vi "PH_SSAC.Draw GUI Image.vi"(0 "i ref in":refnum<vi>, 5 "error in":errorcluster) -> (14 "i ref out":refnum<vi>, 19 "error out":errorcluster)   [LabVIEW 2014, in "PH_SSAC.lvlib"]
doc: "This VI draws the image to the GUI."
uses:
  PH_SSAC.lvlib
  PH_Basics/PH_Img_BaseClass/PH_Img_BaseClass.lvlib
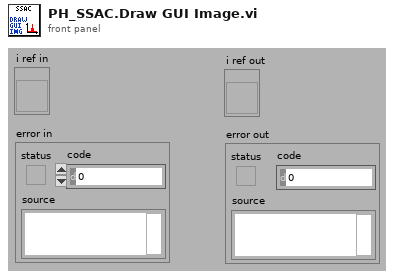
[diagram p1: front panel]
types:
  T1 = typedef "PH_SSAC.lvlib/PH_SSAC.i attribute.ctl" = cluster{"GUI Refs":cluster{"Delete":refnum<vi>, "Global On":refnum<vi>, "Cam Source":refnum<vi>, "Frame Main Signal":refnum<vi>, "Frame Background":refnum<vi>, "dt (Gauss smooth)":refnum<vi>, "Calibration Factor":refnum<vi>, "Background acquire":refnum<vi>, "Threshold":refnum<vi>, "Time evolution of mean pulse duration":refnum<vi>, "Mean Pulse Duration":refnum<vi>, "Main signal":refnum<vi>, "Current Pulse Duration":refnum<vi>, "Processed":refnum<vi>, "Saturation":refnum<vi>, "# for Average":refnum<vi>, "Position":refnum<vi>, "BG Status":refnum<vi>, "Save BG data":refnum<vi>, "Read BG Data":refnum<vi>, "Background Calibration Data":refnum<vi>}, "Images":cluster{"OP Image":T2, "GUI Image":T2, "PSDB Image":T2}, "Global On?":bool, "Frame Main":cluster{"x":u32, "dx":u32, "y":u32, "dy":u32}, "Frame Background":cluster{"x":u32, "dx":u32, "y":u32, "dy":u32}, "dt [fs]":dbl, "Calibration Factor [fs/pixel]":dbl, "Threshold":dbl, "Time evolution of mean pulse duration [fs]":dbl[], "Main Signal":cluster{"Time for Main":dbl[], "Signal":dbl[]}, "Processed":bool, "Current Pulse Duration [fs]":dbl, "# for Average":i32, "Position":i32, "Pulse Durations [fs]":dbl[], "BG":cluster{"Acquire?":bool, "Background Calibration Data":T3, "Save Data":bool}}
  T2 = typedef "IMAQ Image.ctl" = refnum<image>
  T3 = typedef "PH_SSAC.lvlib/PH_SSAC.Background Data.ctl" = cluster{"Date":string, "Time":string, "Frame Main":cluster{"x":u32, "dx":u32, "y":u32, "dy":u32}, "dt [fs]":dbl, "Calibration Factor [fs/pixel]":dbl, "Signal":dbl[], "Frame Background":cluster{"x":u32, "dx":u32, "y":u32, "dy":u32}}
  T4 = cluster{"Left":i32, "Top":i32, "Right":i32, "Bottom":i32}
  T5 = typedef "PH_Img_BaseClass.lvlib/PH_Img_BaseClass.i attribute.ctl" = cluster{"GUI Refs":T6, "Timeout Image [ms]":i32, "Default Periodic Period [ms]":i32, "Camera":cluster{"Instancename":string, "Notifier":refnum<notifier>}, "Palette":T7, "Cam Settings":cluster{"Cam ID":string, "Gain":dbl, "Brightness":dbl, "Shutter":dbl, "Cam Info Failure":bool, "Mode":i32}}
  T6 = typedef "PH_Img_BaseClass.lvlib/PH_Img_BaseClass.GUI Refs.ctl" = cluster{"Timeout":refnum<vi>, "Image":refnum<vi>, "Palette":refnum<vi>, "Timeout Set":refnum<vi>}
  T7 = typedef "PH_Img_BaseClass.lvlib/PH_Img_BaseClass.Palette.ctl" = i32
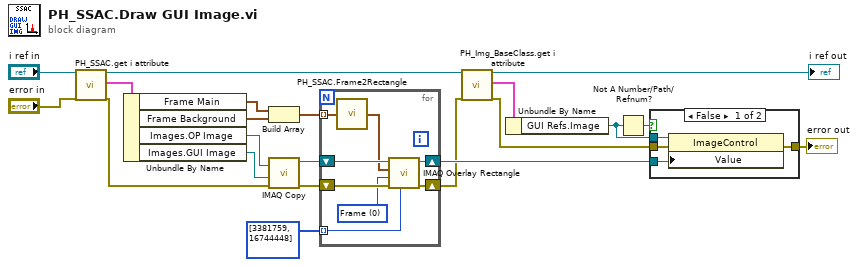
[diagram p0: block diagram]
diagram:
  n1 = call "PH_SSAC.get i attribute.vi"("i ref in"="i ref in", "error in (no error)"="error in") -> ("i ref out"=w19:refnum<vi>, "i attribute"=w20:T1, "error out"=w6:errorcluster)  [unwired: 15 in]
  n2 = Unbundle By Name(w20) -> ("Frame Main"=w10:cluster{"x":u32, "dx":u32, "y":u32, "dy":u32}, "Frame Background"=w9:cluster{"x":u32, "dx":u32, "y":u32, "dy":u32}, "Images.OP Image"=w16:T2, "Images.GUI Image"=w15:T2)
  n3 = Build Array(w10, w9) -> (w8:cluster{"x":u32, "dx":u32, "y":u32, "dy":u32}[])
  n4 = call "IMAQ Copy"("error in (no error)"=w6, "Image Dst"=w15, "Image Src"=w16) -> ("error out"=w14:errorcluster, "Image Dst Out"=w13:T2)  [unwired: 3 in]
  n5 = for {
    shift-right: [w26] -> w12
    shift-left: w13 -> [w27]
    shift-right: [w28] -> w4
    shift-left: w14 -> [w29]
    tunnel: w8 -> [w24] mode=indexing
    tunnel: u32[] [3381759, 16744448] -> [w23] mode=indexing
    w22 = u32 0 items=["Frame", "Fill", "Highlight"] ("Drawing Mode (Frame)")
    n6 = call "PH_SSAC.Frame2Rectangle.vi"("Frame"=w24) -> ("Rectangle"=w25:T4)
    n7 = call "IMAQ Overlay Rectangle"("Color"=w23, "error in (no error)"=w29, "Drawing Mode (Frame)"=w22, "Rectangle"=w25, "Image"=w27) -> ("error out"=w28:errorcluster, "Image Out"=w26:T2)  [unwired: 5 in]
  }
  n8 = call "PH_Img_BaseClass.get i attribute.vi"("i ref in"=w19, "error in (no error)"=w4) -> ("i ref out"=→"i ref out":refnum<vi>, "i attribute"=w2:T5, "error out"=w3:errorcluster)  [unwired: 15 in]
  n9 = Unbundle By Name(w2) -> ("GUI Refs.Image"=w1:refnum<vi>)
  n10 = Not A Number/Path/Refnum?(number/path/refnum=w1) -> (NaN/Path/Refnum?=w21:bool)
  n11 = case shown="False" w21 {
    tunnel: w1 -> [w33 _]
    tunnel: [w32 w34] -> w11
    tunnel: w12 -> [w31 _]
    tunnel: w3 -> [w30 w34]
    frame False {
      n12 = property class="ImageControl"(reference=w33, error in=w30, "Value"=w31) -> (error out=w32:errorcluster)  [unwired: 1 out]
    }
    frame True {
    }
  }
  "error out" <- w11
